vi "Run greeter_server.vi"() -> ()   [LabVIEW 2019, in "helloworld_server.lvlib"]
uses:
  helloworld_server.lvlib
  labview source/gRPC lv Servicer/Servicer/Servicer.lvclass
  RPC Service/Greeter/Greeter.lvclass
panel:
  in  "error in":errorcluster
  out "error out":errorcluster
  out "Listening Port":i32
  in  "Stop":bool
  in  "Server Address":string="localhost:50051"
  in  "Server Certificate File (.crt)":path
  in  "Server Key File (.key)":path
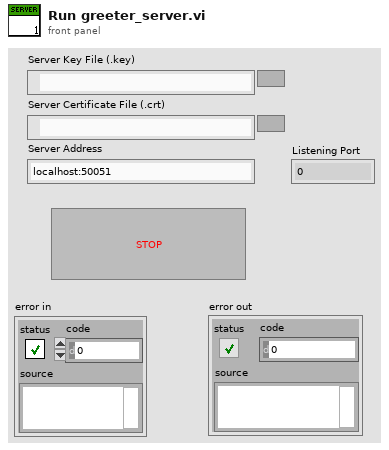
[diagram p1: front panel]
types:
  T1 = typedef "grpc-lvsupport.lvlib/grpcId.ctl" = u64
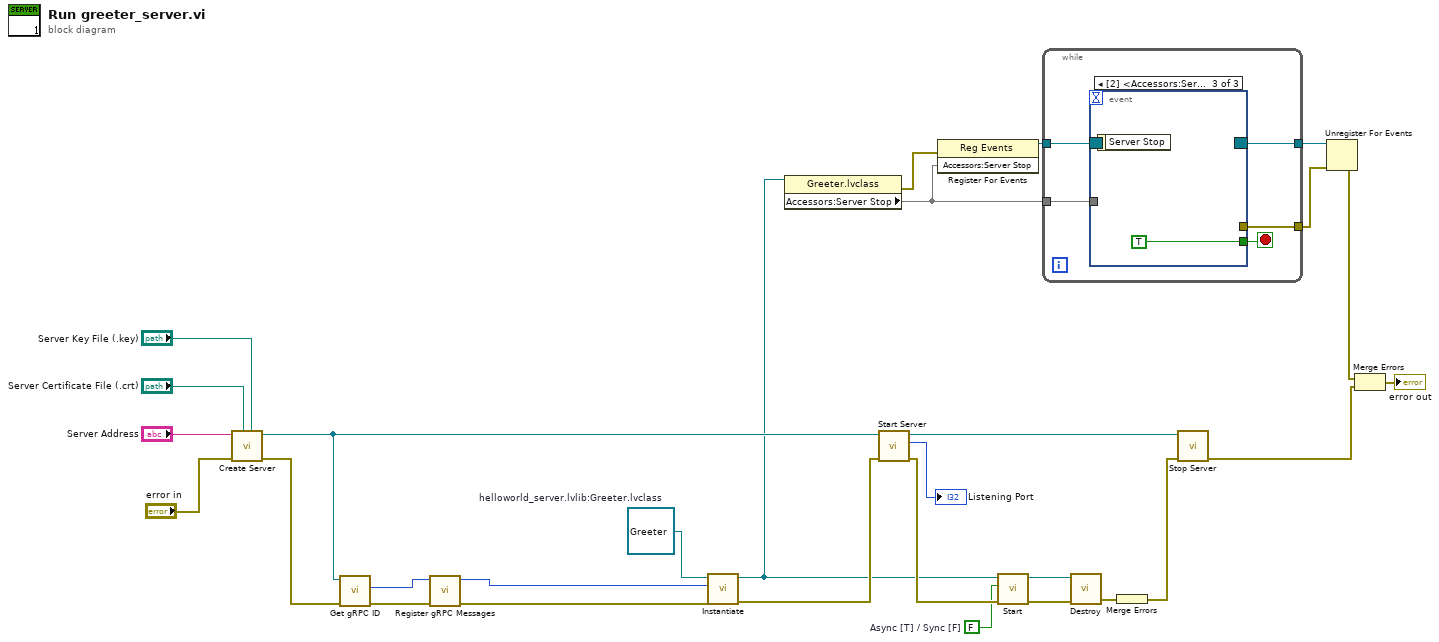
[diagram p0: block diagram]
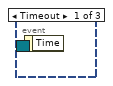
[diagram p2: hidden frame]
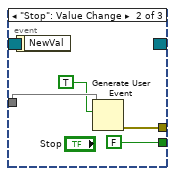
[diagram p3: hidden frame]
diagram:
  w10 = FALSE  # Async [T] / Sync [F]
  w7 = refnum<class "Greeter.lvclass"> refnum  # helloworld_server.lvlib:Greeter.lvclass
  n1 = call "Create Server.vi"("Server Key File (.key)"="Server Key File (.key)", "Server Certificate File (.crt)"="Server Certificate File (.crt)", "error in"="error in", "Server Address"="Server Address") -> ("error out"=w2:errorcluster, "gRPC Server out"=w22:refnum<class "Servicer.lvclass">)  [unwired: 6 in]
  n2 = call "Get gRPC ID.vi"("error in (no error)"=w2, "gRPC Server in"=w22) -> ("error out"=w1:errorcluster, "gRPC ID"=w16:T1)  [unwired: 7 in, 1 out]
  n3 = call "Register gRPC Messages.vi"("error in (no error)"=w1, "gRPC ID"=w16) -> ("error out"=w15:errorcluster, "gRPC ID Out"=w14:T1)  [unwired: 8 in]
  n4 = call-dynamic "Instantiate.vi"("error in"=w15, "gRPCid"=w14, "iService"=w7) -> ("error out"=w20:errorcluster, "iService"=w9:refnum<class "Greeter.lvclass">)  [unwired: 7 in]
  n5 = property class="Greeter.lvclass"(reference=w9) -> (error out=w21:errorcluster, "Accessors:Server Stop"=w8)  [unwired: 1 in, 1 out]
  n6 = call "Start Server.vi"("error in"=w20, "gRPC Server in"=w22) -> ("error out"=w13:errorcluster, "Listening Port"=→"Listening Port":i32, "gRPC Server out"=w29:refnum<class "Servicer.lvclass">)  [unwired: 7 in]
  n7 = register-events(error in=w21, w8) -> (reference out=w25:refnum<event-registration>)  [unwired: 1 in, 1 out]
  n8 = call-dynamic "Start.vi"("error in"=w13, "ASync [T]"=w10, "iService in"=w9) -> ("error out"=w12:errorcluster, "iService out"=w11:refnum<class "Greeter.lvclass">)  [unwired: 7 in]
  n9 = while {
    tunnel: w25 -> [w34]
    tunnel: [w32] -> w24
    tunnel: [w30] -> w17
    tunnel: w8 -> [w31]
    stop <- w33 stop-if-true
    n10 = event shown="[2] <Accessors:Server Stop>: User Event" {
      selector: w34 -> [_ _ _]
      dyn-events: [_ _ _] -> w32
      timeout: _ -> [_ _ _]
      tunnel: [_ FALSE TRUE] -> w33
      tunnel: w31 -> [_ w37 _]
      tunnel: [_ w35 _] -> w30
      event Timeout {
        n11 = event-data() -> ()  [unwired: 1 in, 1 out]
      }
      event "Stop": Value Change {
        n12 = event-data() -> ()  [unwired: 1 in, 1 out]
        n13 = Generate User Event(user event=w37, event data cluster=TRUE ("event data")) -> (error out=w35:errorcluster)  [unwired: 2 in, 1 out]
      }
      event User Event {
        n14 = event-data() -> ()  [unwired: 1 in, 1 out]
      }
    }
  }
  n15 = call-dynamic "Destroy.vi"("error in (no error)"=w12, "SignalGeneratorService in"=w11) -> ("error out"=w19:errorcluster)  [unwired: 8 in, 1 out]
  n16 = Merge Errors(w19) -> (w18:errorcluster)
  n17 = call "Stop Server.vi"("error in"=w18, "gRPC Server in"=w29) -> ("error out"=w6:errorcluster)  [unwired: 9 in]
  n18 = Unregister For Events(event registration refnum=w24, error in=w17) -> (error out=w5:errorcluster)
  n19 = Merge Errors(w5, w6) -> (→"error out":errorcluster)
